vi "PROJECT1_2NDLABVIEW.vi"() -> ()   [LabVIEW 2025]
panel:
  out "LOW":bool
  out "GOOD":bool
  out "HIGH":bool
  in  "Relative Humidity":dbl(slide) scale=0.0..10.0 scale format="%0#1_1f"
  in  "RSens(kOhms)":dbl(slide) scale=0.0..10.0 scale format="%0#1_4f"
  in  "V+":dbl(slide) scale=0.0..10.0 scale format="%0#1_4g"
  in  "Vdiff":dbl(slide) scale=0.0..10.0 scale format="%0#1_4f"
  in  "V_SCC":dbl(slide) scale=0.0..10.0 scale format="%0#1_4f"
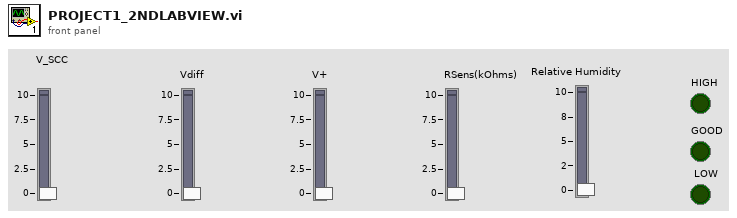
[diagram p1: front panel]
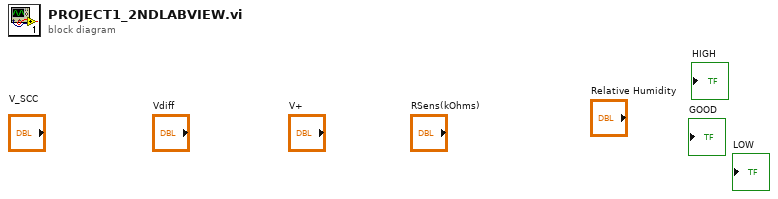
[diagram p0: block diagram]
diagram:
